vi "Write ID.vi"(8 "error in (no error)":errorcluster, 10 "ID":string, 11 "Velodyne 3D LIDAR in":refnum<class "Velodyne 3D LIDAR.lvclass">) -> (0 "error out":errorcluster, 3 "Velodyne 3D LIDAR out":refnum<class "Velodyne 3D LIDAR.lvclass">)   [LabVIEW 2017, in "NI_Robotics_Simulator.lvlib" / "Velodyne 3D LIDAR.lvclass"]
uses:
  <vilib>/robotics/Simulator/Plugin/Sensor/Velodyne 3D LIDAR/Velodyne 3D LIDAR.lvclass
  <vilib>/robotics/Simulator/Plugin/Sensor/Velodyne 3D LIDAR/Velodyne 3D LIDAR.lvclass/Velodyne 3D LIDAR.ctl
  <vilib>/robotics/Simulator/Robot Factory/Sensor/Base/ODESimulator_Base_Sensor.lvclass
  <vilib>/robotics/Simulator/Robot Factory/Joint/ODESimulator_Joint.lvclass
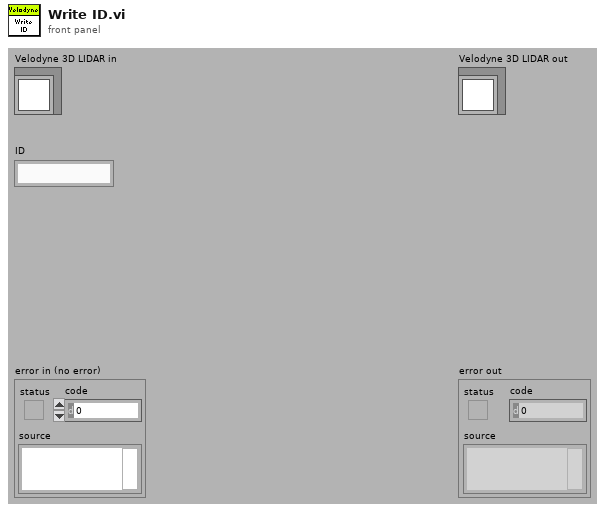
[diagram p1: front panel]
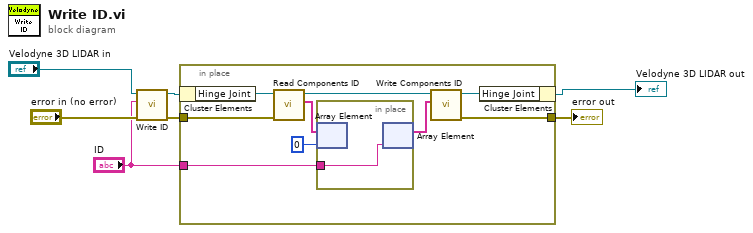
[diagram p0: block diagram]
diagram:
  n1 = call-parent "Write ID.vi"("error in (no error)"="error in (no error)", "ID"="ID", "ODESimulator_Base_Sensor in"="Velodyne 3D LIDAR in") -> ("error out"=w3:errorcluster, "ODESimulator_Base_Sensor out"=w5:refnum<class "Velodyne 3D LIDAR.lvclass">)  [unwired: 7 in]
  n2 = in-place {
    in-place-border: "ID" -> [w13]
    in-place-border: w3 -> [w9]
    in-place-border: [w8] -> w2
    n3 = in-place-cluster #1(w5) -> ("Hinge Joint"=w16:refnum<class "ODESimulator_Joint.lvclass">)
    n4 = call-dynamic "Read Components ID.vi"("error in (no error)"=w9, "Joint in"=w16) -> ("Components ID"=w15:string[], "Joint out"=w12:refnum<class "ODESimulator_Joint.lvclass">)  [unwired: 7 in, 1 out]
    n5 = in-place {
      in-place-border: w13 -> [w17]
      n6 = in-place-array #2(w15, 0) -> ()  [unwired: 1 out]
      n7 = in-place-array #2(w17) -> (w11:string[])  [unwired: 1 out]
    }
    n8 = call-dynamic "Write Components ID.vi"("Components ID"=w11, "Joint in"=w12) -> ("error out"=w8:errorcluster, "Joint out"=w10:refnum<class "ODESimulator_Joint.lvclass">)  [unwired: 8 in]
    n9 = in-place-cluster #1("Hinge Joint"=w10) -> (→"Velodyne 3D LIDAR out":refnum<class "Velodyne 3D LIDAR.lvclass">)
  }
  "error out" <- w2
